vi "OptLobeGuts.vi"(0 "Boolean":bool, 1 "source":string, 2 "Image Out":T1, 4 "error in (no error)":errorcluster, 5 "Array":i16[][](array[numeric]), 7 "New Image":T1, 8 "Session Out":T3, 9 "Image Dst":T1) -> (14 "World":T1, 15 "Working Image":T1(plugin-control), 16 "Boat":T2, 17 "Occupancy Grid":T1(plugin-control), 18 "x":sgl[](array[numeric]), 19 "Buoy 2":cluster{"x":sgl, "y":sgl}, 20 "OccupancyGrid (Raw Data)":i8[][](array[numeric]), 21 "error out":errorcluster, 23 "Bouy 1":cluster{"x":sgl, "y":sgl}, 24 "Nothing":cluster{"x":sgl, "y":sgl}, 25 "Boat":T2, 26 "Dock":cluster{"x":sgl, "y":sgl}, 27 "y":sgl[](array[numeric]))   [LabVIEW 2011]
uses:
  WhereAmI.ctl
  <vilib>/vision/Image Controls.llb/IMAQ Image.ctl
  <vilib>/userdefined/High Color/IMAQdx.ctl
  <vilib>/vision/driver/NI_Vision_Acquisition_Software.lvlib
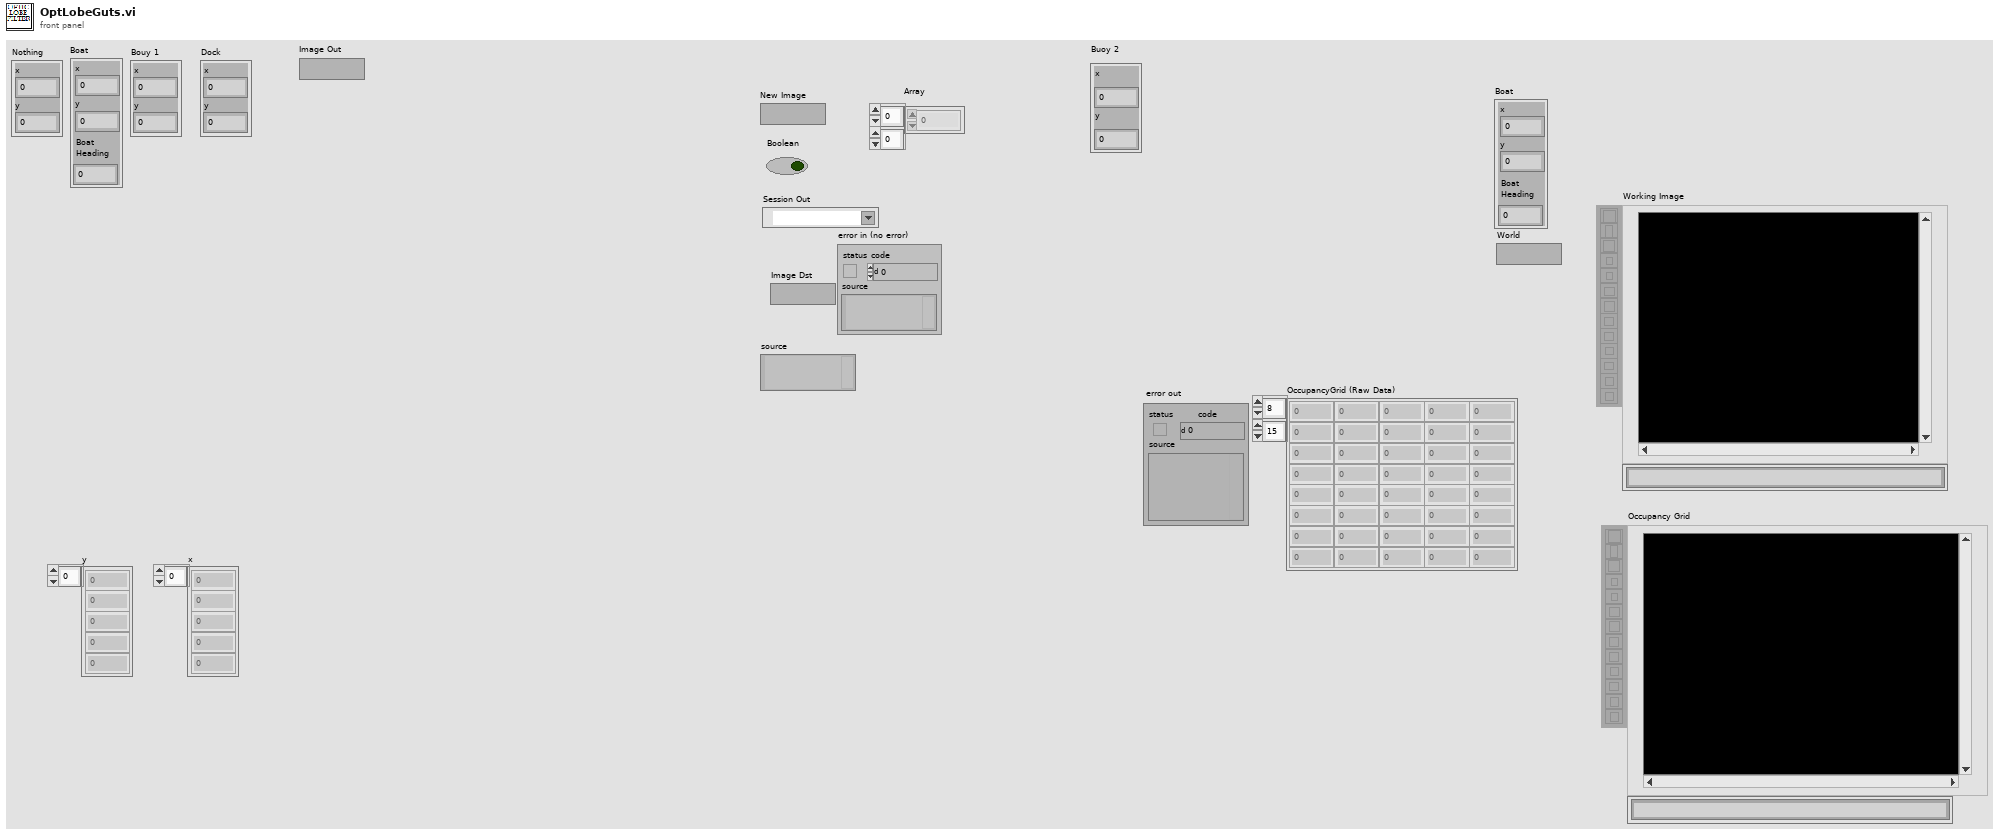
[diagram p1: front panel]
types:
  T1 = typedef "IMAQ Image.ctl" = refnum<image>
  T2 = typedef "WhereAmI.ctl" = cluster{"x":sgl, "y":sgl, "Boat\nHeading":sgl}
  T3 = typedef "IMAQdx.ctl" = refnum<k21>
  T4 = typedef "IMAQ GM Match Report.ctl" = cluster{"Position":cluster{"x":sgl, "y":sgl}, "Angle":sgl, "Scale":sgl, "Score":sgl, "Bounding Box":cluster{"x":sgl, "y":sgl}[], "Contrast Reversed":bool, "Occlusion %":sgl, "Template Target Curve Score":sgl, "Target Template Curve Score":sgl, "Correlation Score":sgl}
  T5 = cluster{"Position":cluster{"x":sgl, "y":sgl}, "Angle":sgl, "Scale":sgl, "Score":sgl, "Bounding Box":cluster{"x":sgl, "y":sgl}[]}[]
  T6 = cluster{"Position":cluster{"x":sgl, "y":sgl}, "Angle":sgl, "Scale":sgl, "Score":sgl, "Bounding Box":cluster{"x":sgl, "y":sgl}[]}
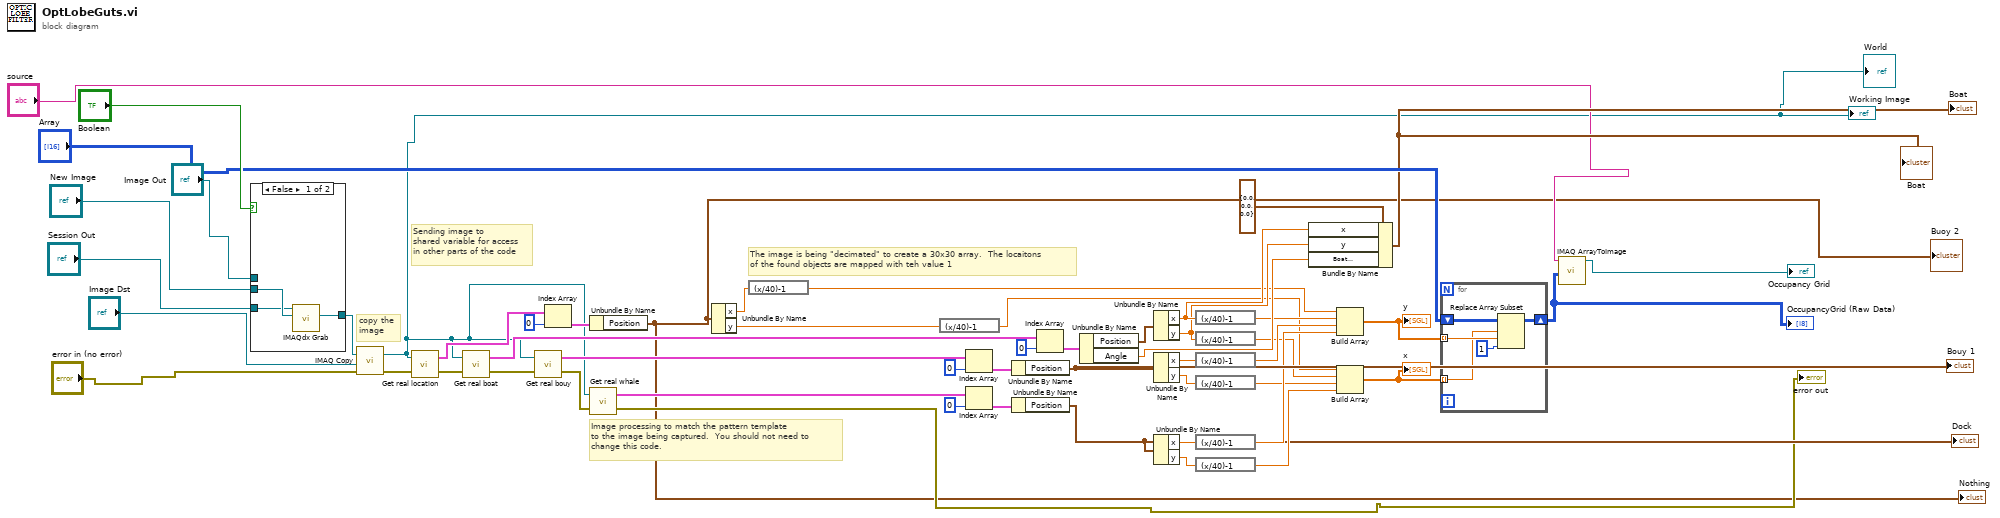
[diagram p0: block diagram]
diagram:
  # "Sending image to\nshared variable for access\nin other parts of the code"
  # "The image is being \"decimated\" to create a 30x30 array.  The locaitons\nof the found objects are mapped with teh value 1"
  # "Image processing to match the pattern template\nto the image being captured.  You should not need to\nchange this code."
  # "copy the\nimage"
  n1 = case shown="False" "Boolean" {
    tunnel: "New Image" -> [w57 _]
    tunnel: "Session Out" -> [w56 _]
    tunnel: "Image Out" -> [_ w58]
    tunnel: [w55 w58] -> w38
    frame False {
      n2 = call <vilib>:"IMAQdx Grab.vi"("Image In"=w57, "Session In"=w56) -> ("Image Out"=w55:T1)  [unwired: 2 in, 7 out]
    }
    frame True {
    }
  }
  n3 = call "IMAQ Copy"("error in (no error)"="error in (no error)", "Image Dst"="Image Dst", "Image Src"=w38) -> ("error out"=w40:errorcluster, "Image Dst Out"=w2:T1)  [unwired: 3 in]
  "Working Image" <- w2
  "World" <- w2
  n4 = call "Get real location.vi"("error in"=w40, "Image"=w2) -> ("error out"=w52:errorcluster, "Matches"=w53:T4[])
  n5 = call "Get real boat.vi"("error in"=w52, "Image"=w2) -> ("error out"=w47:errorcluster, "Matches"=w48:T4[])
  n6 = call "Get real bouy.vi"("error in"=w47, "Image"=w2) -> ("error out"=w43:errorcluster, "Matches"=w44:T4[])
  n7 = Index Array(array=w53, index=0) -> (element=w54:T4)
  n8 = Unbundle By Name(w54) -> ("Position"=w1:cluster{"x":sgl, "y":sgl})
  "Nothing" <- w1
  "Buoy 2" <- w1
  n9 = call "Get real whale.vi"("error in"=w43, "Image"=w2) -> ("error out"=→"error out":errorcluster, "Matches"=w39:T5)
  n10 = Unbundle By Name(w1) -> ("x"=w34:sgl, "y"=w33:sgl)
  n11 = expression code="(x/40)-1"(w34) -> (w25:sgl)
  n12 = expression code="(x/40)-1"(w33) -> (w21:sgl)
  n13 = Index Array(array=w44, index=0) -> (element=w45:T4)
  n14 = Index Array(array=w39, index=0) -> (element=w42:T6)
  n15 = Unbundle By Name(w45) -> ("Position"=w30:cluster{"x":sgl, "y":sgl})
  "Bouy 1" <- w30
  n16 = Unbundle By Name(w42) -> ("Position"=w15:cluster{"x":sgl, "y":sgl})
  "Dock" <- w15
  n17 = Index Array(array=w48, index=0) -> (element=w50:T4)
  n18 = Unbundle By Name(w50) -> ("Position"=w37:cluster{"x":sgl, "y":sgl}, "Angle"=w36:sgl)
  n19 = Unbundle By Name(w37) -> ("x"=w32:sgl, "y"=w31:sgl)
  n20 = Unbundle By Name(w30) -> ("x"=w29:sgl, "y"=w28:sgl)
  n21 = Unbundle By Name(w15) -> ("x"=w27:sgl, "y"=w26:sgl)
  n22 = expression code="(x/40)-1"(w32) -> (w24:sgl)
  n23 = expression code="(x/40)-1"(w31) -> (w20:sgl)
  n24 = expression code="(x/40)-1"(w29) -> (w23:sgl)
  n25 = expression code="(x/40)-1"(w28) -> (w19:sgl)
  n26 = expression code="(x/40)-1"(w27) -> (w22:sgl)
  n27 = expression code="(x/40)-1"(w26) -> (w18:sgl)
  n28 = Bundle By Name(cluster=T2 {"x"=0.0, "y"=0.0, "Boat\nHeading"=0.0} ("Boat"), "x"=w32, "y"=w31, "Boat\nHeading"=w36) -> (→"Boat" →"Boat":T2)
  n29 = Build Array(w25, w24, w23, w22) -> (w17:sgl[])
  "y" <- w17
  n30 = Build Array(w21, w20, w19, w18) -> (w16:sgl[])
  "x" <- w16
  n31 = for {
    tunnel: w17 -> [w62] mode=indexing
    tunnel: w16 -> [w61] mode=indexing
    shift-right: [w59] -> w5
    shift-left: "Array" -> [w63]
    n32 = Replace Array Subset(array=w63, new element=i8 1 ("new element/subarray"), index (row)=w61, index (col)=w62) -> (w59:i16[][])
  }
  "OccupancyGrid (Raw Data)" <- w5
  n33 = call "IMAQ ArrayToImage"("Image Pixels (I16)"=w5, "Image"="source") -> ("Image Out"=→"Occupancy Grid":T1)  [unwired: 8 in, 1 out]
